vi "Pre Launch Init.vi"(11 "Root Tester in":refnum<class "Root Tester.lvclass">) -> (0 "error out":errorcluster, 3 "Root Tester out":refnum<class "Root Tester.lvclass">)   [LabVIEW 2024, in "Root Tester.lvlib" / "Root Tester.lvclass"]
doc: "<p>(<strong>Filename</strong>: <span class=\"dnl\">Actor Framework.lvlib:Actor.lvclass:Pre Launch Init.vi</span>)</p>\n<p>Defines behavior that occurs after the <a href=\"nihelplauncher://docs/csh?context=lvcore_lvcomm_af_launch_nested_actor\">Launch Nested Actor</a> method is invoked but before the actor's Actor Core method begins running.</p>\n<p>By default, this method does nothing. A descendant class may override it to define behavior.</p>"
uses:
  Root Tester.lvclass
  Root Tester.lvclass/Root Tester.ctl
  <vilib>/ActorFramework/Actor/Actor.lvclass
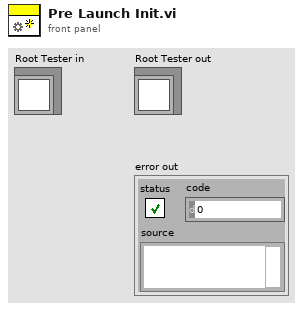
[diagram p1: front panel]
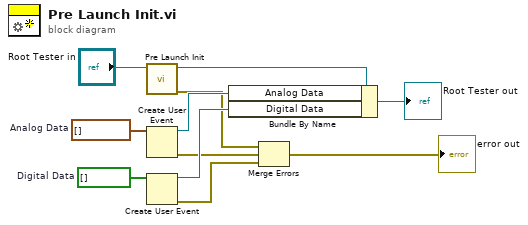
[diagram p0: block diagram]
diagram:
  w7 = waveform(dbl)[] []  # Analog Data
  w10 = bool[] []  # Digital Data
  n1 = call-parent "Pre Launch Init.vi"("Actor in"="Root Tester in") -> ("error out"=w4:errorcluster, "Actor out"=w9:refnum<class "Root Tester.lvclass">)  [unwired: 9 in]
  n2 = Create User Event(user event datatype=w7) -> (user event=w6:refnum<user-event>, error out=w3:errorcluster)  [unwired: 1 in]
  n3 = Create User Event(user event datatype=w10) -> (user event=w5:refnum<user-event>, error out=w2:errorcluster)  [unwired: 1 in]
  n4 = Bundle By Name(cluster=w9, "Analog Data"=w6, "Digital Data"=w5) -> (→"Root Tester out":refnum<class "Root Tester.lvclass">)
  n5 = Merge Errors(w4, w3, w2) -> (→"error out":errorcluster)
